vi "CV_measure_LCR.vi"(0 "Input parameters":T2={"Measurement type"=enum."Debug", "Sensor type"=enum."HPK_8in_271ch", "Identifier"="test.txt", "Open after execution?"=FALSE, "Plot after execution?"=FALSE, "Display channel"=0, "Voltage Delay (s)"=0.5, "Switch Delay (s)"=0.01, "VISA resource name source"="", "VISA resource name DMM"="", "VISA resource name LCR"="", "Compliance  Level (A)"=10.0, "Voltage Limit (V)"=1000.0, "Data storage location"="", "Scan voltages"="", "Use source as DMM?"=FALSE, "LCR signal frequenzy (Hz)"=10.0, "DMM device"=enum."Keithley2001", "Sampling number"=1, "Use env. sensors on"=enum."Sensirion sht1x/7x", "Switchboard Handle"=0, "Use Switchboard"=FALSE, "LCR signal voltage (V)"=10000.0, "Repeat"=1, "Scan voltages IV"="", "Scan voltages CV"="", "Hex pad numbers?"=FALSE, "Set measurement type"=enum."Debug", "Custom pad scan"="", "IV voltage Delay (s)"=0.5, "CV voltage Delay (s)"=0.5, "Needle measurement?"=FALSE, "Comments"="test.txt", "LCR signal frequenzy (kHz)"=10.0, "Compliance  Level (uA)"=10.0, "Open Correction Array"=array2304x3[6912 elements], "Current set voltage"=0.0, "Last set voltage"=0.0, "Current channel"=0, "Last OpenCorrection index"=-1, "Total curr/vltg every x steps"=10, "Current channel iteration"=0, "No CV corrections"=FALSE, "Mapfile"="", "Corrfile"="", "IV voltage file"=path "", "CV voltage file"=path "", "IV Switch Delay (s)"=0.01, "CV Switch Delay (s)"=0.01, "Invert polarity"=FALSE, "Set debug dirs"=FALSE, "Is n on p"=FALSE, "Source interlock?"=TRUE, "Voltage file used?"=FALSE, "Pad mask"="", "Mask pad above (uA)"=1.0, "LCR device"=enum."LCR_E4980", "Source device"=enum."Source_2410", "HexPlot binary path"="", "PadReductionFactor"=1.0, "Temperature degC"="", "Fluence [neq]"="", "Annealing [min]"=""} {"CV Switch Delay (s)" format="%#_13g"; "IV Switch Delay (s)" format="%#_13g"; "Last set voltage" format="%#_13g"; "Current set voltage" format="%#_13g"; "CV voltage Delay (s)" format="%#_13g"; "IV voltage Delay (s)" format="%#_13g"; "Voltage Limit (V)" format="%#_13g"; "Voltage Delay (s)" format="%#_13g"; "Switch Delay (s)" format="%#_13g"}, 11 "error in (no error)":errorcluster) -> (4 "Input parameters out":T2={"Measurement type"=enum."Debug", "Sensor type"=enum."HPK_8in_271ch", "Identifier"="test.txt", "Open after execution?"=FALSE, "Plot after execution?"=FALSE, "Display channel"=0, "Voltage Delay (s)"=0.5, "Switch Delay (s)"=0.01, "VISA resource name source"="", "VISA resource name DMM"="", "VISA resource name LCR"="", "Compliance  Level (A)"=10.0, "Voltage Limit (V)"=1000.0, "Data storage location"="", "Scan voltages"="", "Use source as DMM?"=FALSE, "LCR signal frequenzy (Hz)"=10.0, "DMM device"=enum."Keithley2001", "Sampling number"=1, "Use env. sensors on"=enum."Sensirion sht1x/7x", "Switchboard Handle"=0, "Use Switchboard"=FALSE, "LCR signal voltage (V)"=10000.0, "Repeat"=1, "Scan voltages IV"="", "Scan voltages CV"="", "Hex pad numbers?"=FALSE, "Set measurement type"=enum."Debug", "Custom pad scan"="", "IV voltage Delay (s)"=0.5, "CV voltage Delay (s)"=0.5, "Needle measurement?"=FALSE, "Comments"="test.txt", "LCR signal frequenzy (kHz)"=10.0, "Compliance  Level (uA)"=10.0, "Open Correction Array"=array2304x3[6912 elements], "Current set voltage"=0.0, "Last set voltage"=0.0, "Current channel"=0, "Last OpenCorrection index"=-1, "Total curr/vltg every x steps"=10, "Current channel iteration"=0, "No CV corrections"=FALSE, "Mapfile"="", "Corrfile"="", "IV voltage file"=path "", "CV voltage file"=path "", "IV Switch Delay (s)"=0.01, "CV Switch Delay (s)"=0.01, "Invert polarity"=FALSE, "Set debug dirs"=FALSE, "Is n on p"=FALSE, "Source interlock?"=TRUE, "Voltage file used?"=FALSE, "Pad mask"="", "Mask pad above (uA)"=1.0, "LCR device"=enum."LCR_E4980", "Source device"=enum."Source_2410", "HexPlot binary path"="", "PadReductionFactor"=1.0, "Temperature degC"="", "Fluence [neq]"="", "Annealing [min]"=""} {"CV Switch Delay (s)" format="%#_13g"; "IV Switch Delay (s)" format="%#_13g"; "Last set voltage" format="%#_13g"; "Current set voltage" format="%#_13g"; "CV voltage Delay (s)" format="%#_13g"; "IV voltage Delay (s)" format="%#_13g"; "Voltage Limit (V)" format="%#_13g"; "Voltage Delay (s)" format="%#_13g"; "Switch Delay (s)" format="%#_13g"}, 8 "LCR data":T1, 15 "error out":errorcluster)   [LabVIEW 2020]
doc: "Measure capacitance and connected quantities from LCR meter."
uses:
  input_params.ctl
  data_LCR.ctl
  <instrlib>/Agilent E4980/Agilent E4980.lvlib
  <instrlib>/Agilent 4263X/Agilent 4263X.lvlib
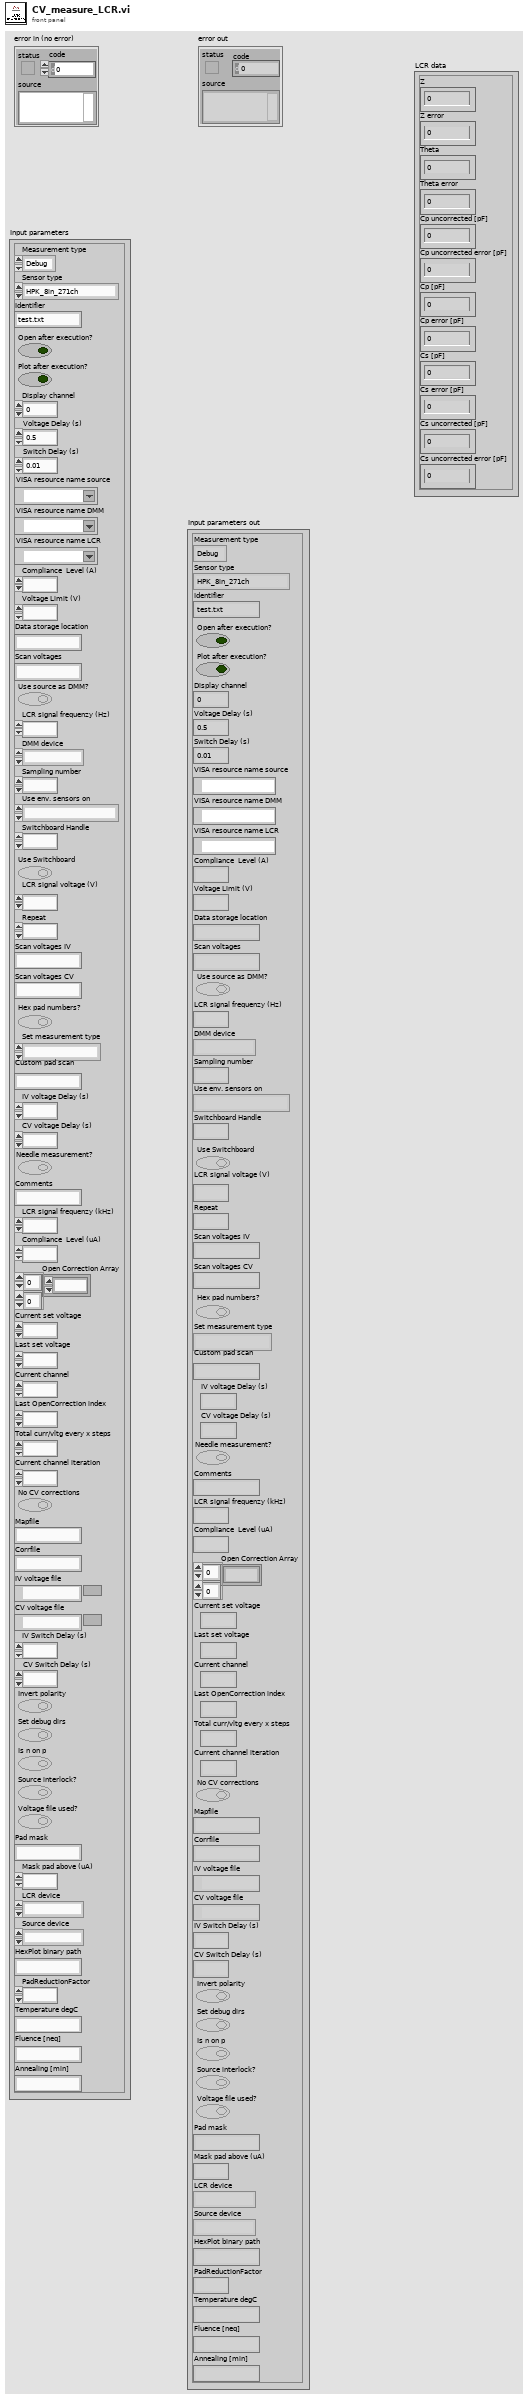
[diagram p1: front panel]
types:
  T1 = typedef "data_LCR.ctl" = cluster{"Z":dbl, "Z error":dbl, "Theta":dbl, "Theta error":dbl, "Cp uncorrected [pF]":dbl, "Cp uncorrected error [pF]":dbl, "Cp [pF]":dbl, "Cp error [pF]":dbl, "Cs [pF]":dbl, "Cs error [pF]":dbl, "Cs uncorrected [pF]":dbl, "Cs uncorrected error [pF]":dbl}
  T2 = typedef "input_params.ctl" = cluster{"Measurement type":enum16{"IV", "CV", "Debug", "Test_contact"}, "Sensor type":enum16{"HPK_6in_135ch", "HPK_8in_271ch", "IFX_8in_256ch", "Diode", "HPK_6in_239ch", "Full_Matrix", "HPK_8in_271ch_full", "LumiCal", "HPK_8in_444ch", "HPK_8in_198ch_2019", "HPK_8in_MGW_LD_full", "HPK_8in_MGW_LD_a_type_top", "HPK_8in_MGW_LD_a_type_bottom", "HPK_8in_MGW_LD_b_type_left", "HPK_8in_MGW_LD_b_type_right", "HPK_8in_MGW_LD_c_type_left", "HPK_8in_MGW_LD_c_type_right", "HPK_8in_MGW_HD_full", "HPK_8in_MGW_HD_a_type_top", "HPK_8in_MGW_HD_a_type_bottom", "HPK_8in_MGW_HD_b_type_left", "HPK_8in_MGW_HD_b_type_right", "HPK_8in_MGW_HD_c_type_left", "HPK_8in_MGW_HD_c_type_right", "CALICE_6in_256ch"}, "Identifier":string, "Open after execution?":bool, "Plot after execution?":bool, "Display channel":i32, "Voltage Delay (s)":dbl, "Switch Delay (s)":dbl, "VISA resource name source":refnum<visa-resource-name>, "VISA resource name DMM":refnum<visa-resource-name>, "VISA resource name LCR":refnum<visa-resource-name>, "Compliance  Level (A)":dbl, "Voltage Limit (V)":dbl, "Data storage location":string, "Scan voltages":string, "Use source as DMM?":bool, "LCR signal frequenzy (Hz)":dbl, "DMM device":enum16{"Keithley2001", "Keithley2450", "Keithley2410", "Keithley6485", "Keithley6487", "Keithley6517"}, "Sampling number":i32, "Use env. sensors on":enum16{"Sensirion sht1x/7x", "Switch Matrix", "Probecard"}, "Switchboard Handle":u32, "Use Switchboard":bool, "LCR signal voltage (V)":dbl, "Repeat":i32, "Scan voltages IV":string, "Scan voltages CV":string, "Hex pad numbers?":bool, "Set measurement type":enum16{"IV", "CV", "Debug", "Test_contact", "IV+CV"}, "Custom pad scan":string, "IV voltage Delay (s)":dbl, "CV voltage Delay (s)":dbl, "Needle measurement?":bool, "Comments":string, "LCR signal frequenzy (kHz)":dbl, "Compliance  Level (uA)":dbl, "Open Correction Array":dbl[][], "Current set voltage":dbl, "Last set voltage":dbl, "Current channel":i32, "Last OpenCorrection index":i32, "Total curr/vltg every x steps":i32, "Current channel iteration":i32, "No CV corrections":bool, "Mapfile":string, "Corrfile":string, "IV voltage file":path, "CV voltage file":path, "IV Switch Delay (s)":dbl, "CV Switch Delay (s)":dbl, "Invert polarity":bool, "Set debug dirs":bool, "Is n on p":bool, "Source interlock?":bool, "Voltage file used?":bool, "Pad mask":string, "Mask pad above (uA)":dbl, "LCR device":enum16{"LCR_E4980", "AGILENT_4263X"}, "Source device":enum16{"Source_2410", "Source_6487", "Source_2470"}, "HexPlot binary path":string, "PadReductionFactor":dbl, "Temperature degC":string, "Fluence [neq]":string, "Annealing [min]":string}
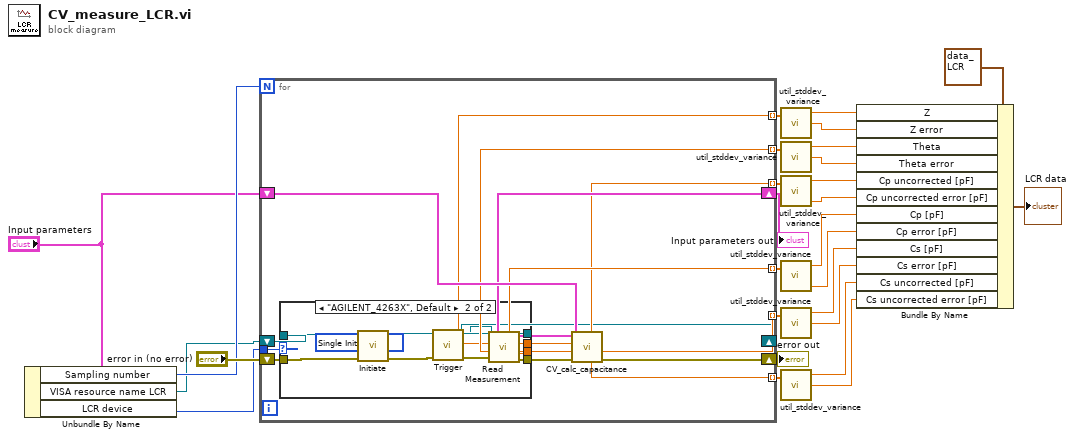
[diagram p0: block diagram]
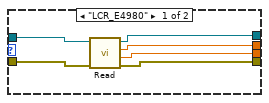
[diagram p2: hidden frame]
diagram:
  n1 = Unbundle By Name("Input parameters") -> ("Sampling number"=w25:i32, "VISA resource name LCR"=w1:refnum<visa-resource-name>, "LCR device"=w2:enum16{"LCR_E4980", "AGILENT_4263X"})
  n2 = for {
    N: w25 -> [_]
    tunnel: [w34] -> w22 mode=indexing
    tunnel: [w33] -> w21 mode=indexing
    tunnel: [w35] -> w24 mode=indexing
    tunnel: [w36] -> w23 mode=indexing
    shift-right: [w39] -> w27
    shift-left: "error in (no error)" -> [w41]
    tunnel: [w32] -> w18 mode=indexing
    tunnel: [w31] -> w17 mode=indexing
    shift-right: [w37] -> w19
    shift-left: "Input parameters" -> [w38]
    tunnel: w2 -> [w30]
    shift-right: [w29] -> _
    shift-left: w1 -> [w28]
    n3 = case shown="\"AGILENT_4263X\", Default" w30 {
      tunnel: w28 -> [w47 w50]
      tunnel: w41 -> [w46 w49]
      tunnel: [w43 w58] -> w40
      tunnel: [w44 w56] -> w36
      tunnel: [w45 w57] -> w35
      tunnel: [w42 w55] -> w29
      frame "LCR_E4980" {
        n4 = call <instrlib>:"Read.vi"("error in (no error)"=w46, "VISA resource name"=w47) -> ("error out"=w43:errorcluster, "Secondary Parameter"=w44:dbl, "Primary Parameter"=w45:dbl, "VISA resource name out"=w42:refnum<visa-resource-name>)  [unwired: 6 in]
      }
      frame "AGILENT_4263X", Default {
        w48 = u16 1 items=["Continuous Initiate", "Single Initiate", "Stop Continuous"] ("initiate mode (0:continuous)")
        n5 = call <instrlib>:"Initiate.vi"("error in (no error)"=w49, "initiate mode (0:continuous)"=w48, "VISA resource name"=w50) -> ("error out"=w51:errorcluster, "VISA resource name out"=w52:refnum<visa-resource-name>)  [unwired: 7 in]
        n6 = call <instrlib>:"Trigger.vi"("error in (no error)"=w51, "VISA resource name"=w52) -> ("error out"=w54:errorcluster, "VISA resource name out"=w53:refnum<visa-resource-name>)  [unwired: 8 in]
        n7 = call <instrlib>:"Read Measurement.vi"("VISA resource name"=w53, "error in (no error)"=w54) -> ("VISA resource name out"=w55:refnum<visa-resource-name>, "primary reading"=w57:dbl, "secondary reading"=w56:dbl, "error out"=w58:errorcluster)  [unwired: 7 in, 3 out]
      }
    }
    n8 = call "CV_calc_capacitance.vi"("error in (no error)"=w40, "Theta (Phase)"=w36, "Z (impedance)"=w35, "Input parameters"=w38) -> ("error out"=w39:errorcluster, "Cs [pF]"=w33:dbl, "Cp [pF]"=w34:dbl, "Input parameters out"=w37:T2, "Cs uncorrected [pF]"=w31:dbl, "Cp uncorrected [pF]"=w32:dbl)  [unwired: 2 in]
  }
  "error out" <- w27
  "Input parameters out" <- w19
  n9 = call "util_stddev_variance.vi"("X"=w24) -> ("mean"=w4:dbl, "standard deviation"=w5:dbl)  [unwired: 1 in, 1 out]
  n10 = call "util_stddev_variance.vi"("X"=w23) -> ("mean"=w3:dbl, "standard deviation"=w6:dbl)  [unwired: 1 in, 1 out]
  n11 = call "util_stddev_variance.vi"("X"=w18) -> ("mean"=w7:dbl, "variance"=w8:dbl)  [unwired: 1 in, 1 out]
  n12 = call "util_stddev_variance.vi"("X"=w22) -> ("mean"=w9:dbl, "variance"=w10:dbl)  [unwired: 1 in, 1 out]
  n13 = call "util_stddev_variance.vi"("X"=w21) -> ("mean"=w11:dbl, "standard deviation"=w12:dbl)  [unwired: 1 in, 1 out]
  n14 = call "util_stddev_variance.vi"("X"=w17) -> ("mean"=w13:dbl, "standard deviation"=w14:dbl)  [unwired: 1 in, 1 out]
  n15 = Bundle By Name(cluster=T1 {"Z"=0.0, "Z error"=0.0, "Theta"=0.0, "Theta error"=0.0, "Cp uncorrected [pF]"=0.0, "Cp uncorrected error [pF]"=0.0, "Cp [pF]"=0.0, "Cp error [pF]"=0.0, "Cs [pF]"=0.0, "Cs error [pF]"=0.0, "Cs uncorrected [pF]"=0.0, "Cs uncorrected error [pF]"=0.0} ("Cluster"), "Z"=w4, "Z error"=w5, "Theta"=w3, "Theta error"=w6, "Cp uncorrected [pF]"=w7, "Cp uncorrected error [pF]"=w8, "Cp [pF]"=w9, "Cp error [pF]"=w10, "Cs [pF]"=w11, "Cs error [pF]"=w12, "Cs uncorrected [pF]"=w13, "Cs uncorrected error [pF]"=w14) -> (→"LCR data":T1)
